vi "2013_01_02 Durability8 Main.vi"() -> ()   [LabVIEW 2011]
uses:
  MotorTypeDef.ctl
  <vilib>/DAQmx/write.llb/DAQmx Write (Counter Time 1Chan 1Samp).vi
  <vilib>/DAQmx/read.llb/DAQmx Read (Analog 1D Wfm NChan NSamp).vi
  <vilib>/Utility/TradDaqScaling.llb/Convert Thermistor Reading (waveform).vi
  <vilib>/DAQmx/miscellaneous.llb/DAQmx Fill In Error Info.vi
  <vilib>/measure/madcrms.llb/Averaged DC-RMS for N Chan.vi
  <vilib>/measure/NI_MAPro.lvlib
panel:
  out "for loop":i32
  out "Saving Data 2":bool caption="Saving Data"
  in  "new_file event":bool caption="new_file"
  out "Saving Data":bool
  in  "Coarse File Path":path=path "Durability/coarse.lvm"
  in  "Fine File Path":path=path "Durability/fine.lvm"
  out "Voltages":waveform(dbl)[](graph)
  out "Currents":waveform(dbl)[](graph)
  in  "Motor 8":T1 {"Elapsed Time" format="%<%H:%M:%S>t"; "Efficiency" format="%#_3g%%"; "Supply Voltage (V)" format="%#_3f"; "Power Output (W)" format="%#_3g"; "Power Usage (W)" format="%#_3g"; "Torque (mNm)" format="%#_3g"; "RPM" scale=0.0..40000.0 scale format="%#.6p"}
  in  "Motor 7":T1 {"Elapsed Time" format="%<%H:%M:%S>t"; "Efficiency" format="%#_3g%%"; "Supply Voltage (V)" format="%#_3f"; "Power Output (W)" format="%#_3g"; "Power Usage (W)" format="%#_3g"; "Torque (mNm)" format="%#_3g"; "RPM" scale=0.0..40000.0 scale format="%#.6p"}
  in  "Motor 6":T1 {"Elapsed Time" format="%<%H:%M:%S>t"; "Efficiency" format="%#_3g%%"; "Supply Voltage (V)" format="%#_3f"; "Power Output (W)" format="%#_3g"; "Power Usage (W)" format="%#_3g"; "Torque (mNm)" format="%#_3g"; "RPM" scale=0.0..40000.0 scale format="%#.6p"}
  in  "Motor 5":T1 {"Elapsed Time" format="%<%H:%M:%S>t"; "Efficiency" format="%#_3g%%"; "Supply Voltage (V)" format="%#_3f"; "Power Output (W)" format="%#_3g"; "Power Usage (W)" format="%#_3g"; "Torque (mNm)" format="%#_3g"; "RPM" scale=0.0..40000.0 scale format="%#.6p"}
  in  "Motor 4":T1 {"Elapsed Time" format="%<%H:%M:%S>t"; "Efficiency" format="%#_3g%%"; "Supply Voltage (V)" format="%#_3f"; "Power Output (W)" format="%#_3g"; "Power Usage (W)" format="%#_3g"; "Torque (mNm)" format="%#_3g"; "RPM" scale=0.0..40000.0 scale format="%#.6p"}
  in  "Motor 3":T1 {"Elapsed Time" format="%<%H:%M:%S>t"; "Efficiency" format="%#_3g%%"; "Supply Voltage (V)" format="%#_3f"; "Power Output (W)" format="%#_3g"; "Power Usage (W)" format="%#_3g"; "Torque (mNm)" format="%#_3g"; "RPM" scale=0.0..40000.0 scale format="%#.6p"}
  in  "Motor 2":T1 {"Elapsed Time" format="%<%H:%M:%S>t"; "Efficiency" format="%#_3g%%"; "Supply Voltage (V)" format="%#_3f"; "Power Output (W)" format="%#_3g"; "Power Usage (W)" format="%#_3g"; "Torque (mNm)" format="%#_3g"; "RPM" scale=0.0..40000.0 scale format="%#.6p"}
  in  "Motor 1":T1 {"Elapsed Time" format="%<%H:%M:%S>t"; "Efficiency" format="%#_3g%%"; "Supply Voltage (V)" format="%#_3f"; "Power Output (W)" format="%#_3g"; "Power Usage (W)" format="%#_3g"; "Torque (mNm)" format="%#_3g"; "RPM" scale=0.0..40000.0 scale format="%#.6p"}
  out "Motor Temp":dbl(slide) scale=90.0..110.0
  out "Tank Temp":dbl(slide) scale=90.0..110.0
  out "RMS Voltages":waveform(dbl)[](graph)
  out "RMS Currents":waveform(dbl)[](graph)
  in  "Temp Probe\nOn Motor":dbl=1.0
  out "loop time (ms)":u32
  in  "stop":bool
  in  "Unlock PWM":bool=TRUE
  in  "PWM 2":dbl(slide)=100.0 min=0.0 max=100.0 step=5.0 scale=0.0..100.0
  in  "PWM 1":dbl(slide) min=0.0 max=100.0 step=5.0 scale=0.0..100.0
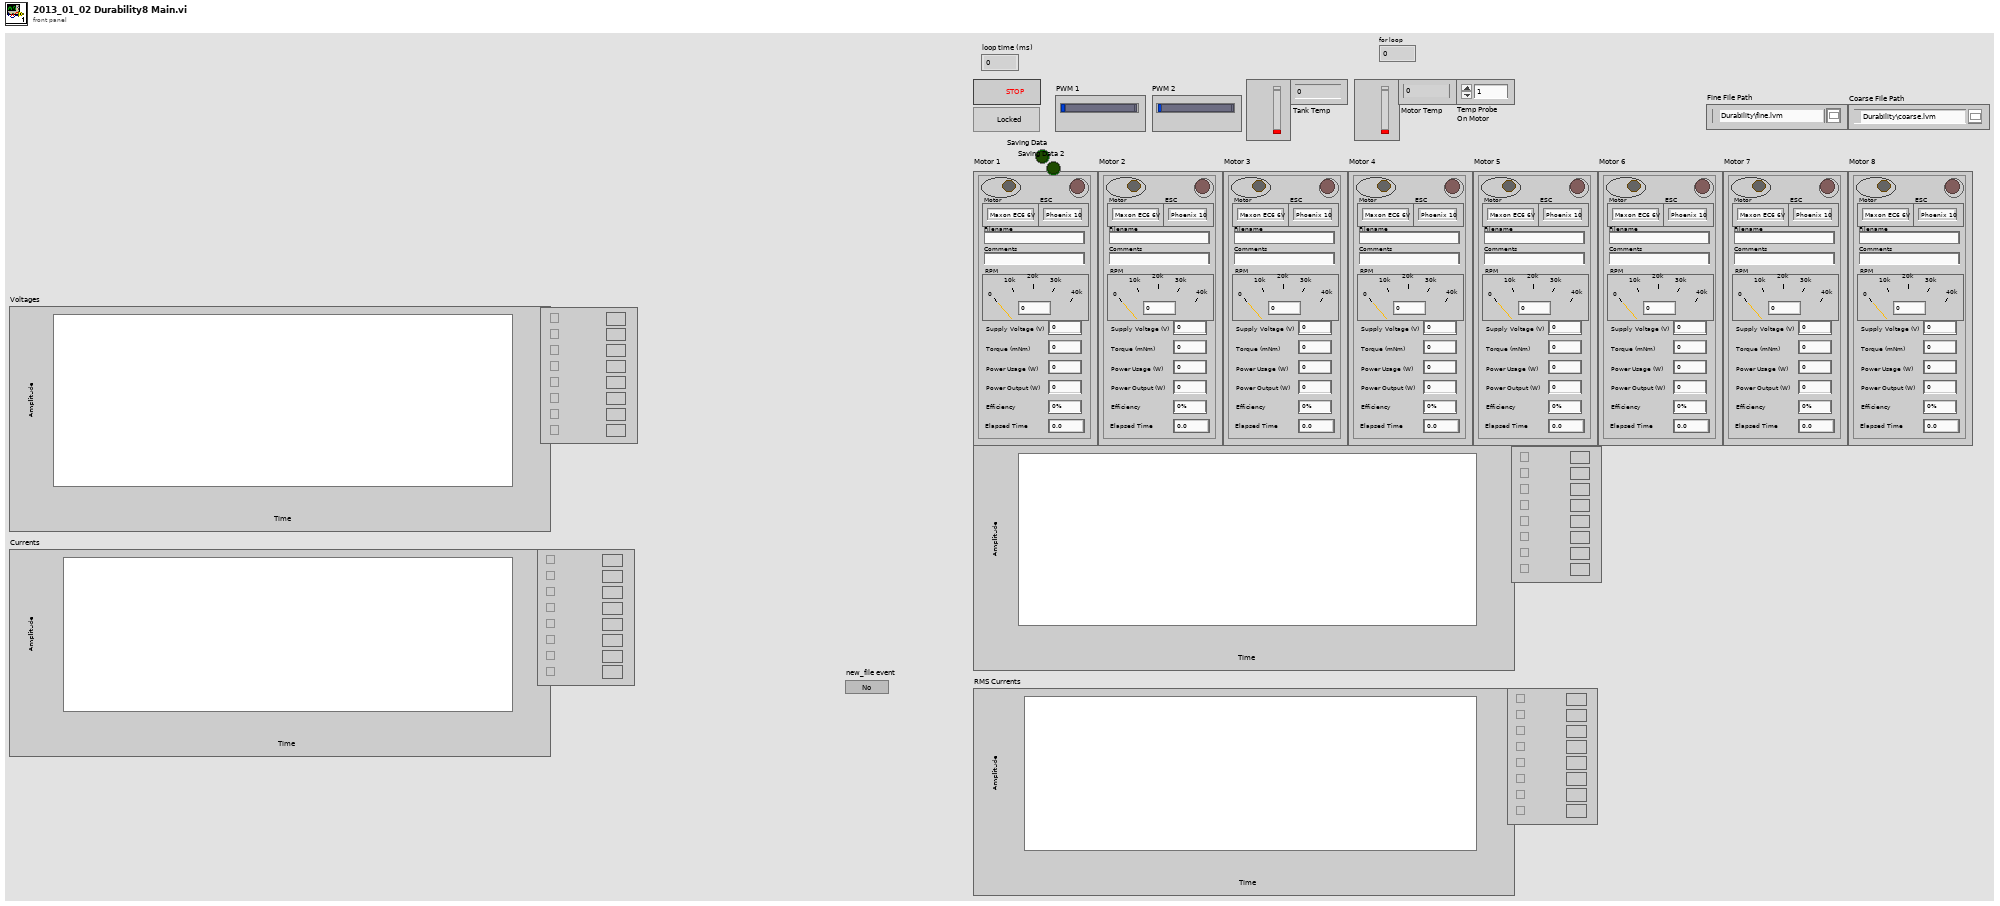
[diagram p1: front panel]
types:
  T1 = typedef "MotorTypeDef.ctl" = cluster{"Enabled":bool, "Fail":bool, "RPM":dbl, "Motor":enum16{"Maxon EC6 6V", "Maxon EC4 6V", "FH 0620 6V", "FH 0620 12V"}, "ESC":enum16{"Phoenix 10", "Maxon", "FH 1801"}, "Torque (mNm)":dbl, "Power Usage (W)":dbl, "Power Output (W)":dbl, "Supply Voltage (V)":dbl, "Efficiency":dbl, "Filename":string, "Comments":string, "Elapsed Time":dbl}
  T2 = enum8{"Enabled", "Disabled", "Disabled and Grayed Out"}
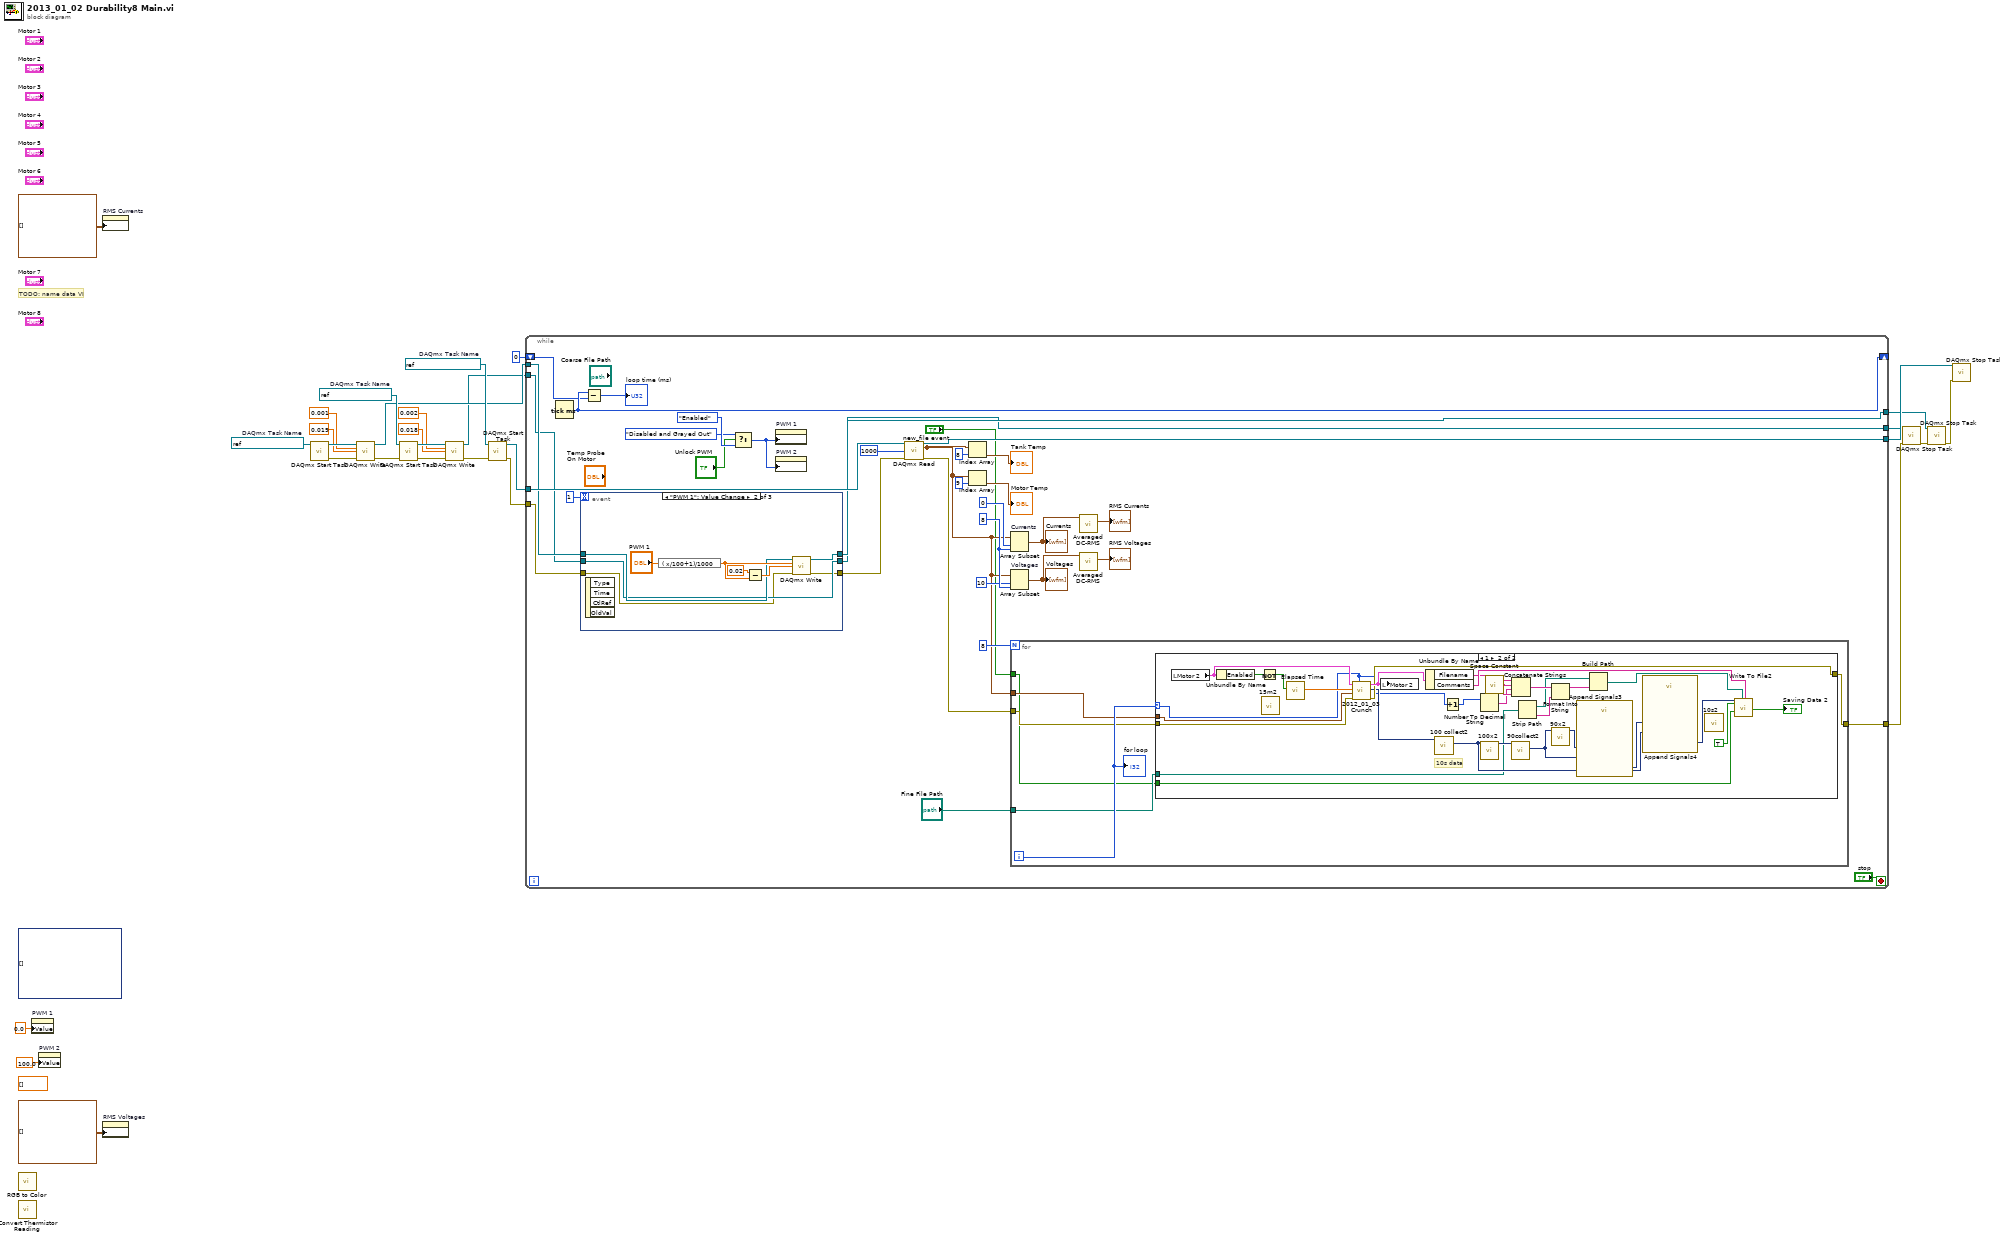
[diagram p0: block diagram]
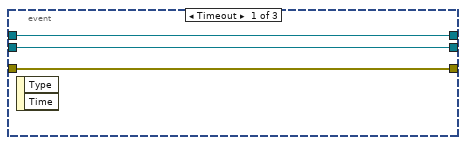
[diagram p2: hidden frame]
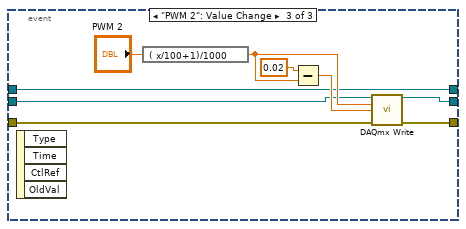
[diagram p3: hidden frame]
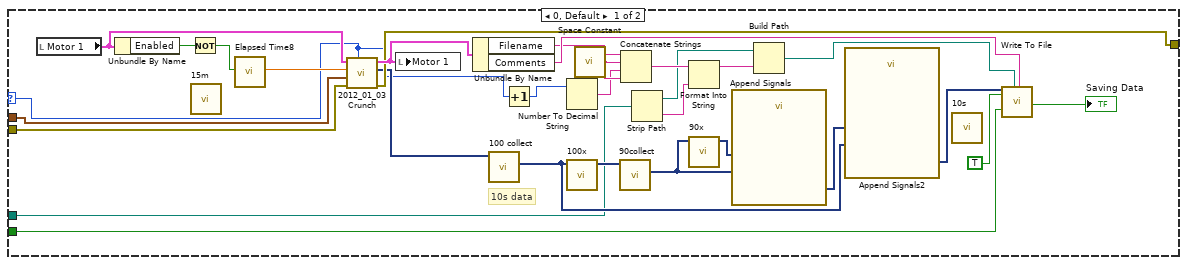
[diagram p4: hidden frame]
diagram:
  (unwired) dynamicdata[] []
  (unwired) dbl[] [] ("History Data")
  w23 = refnum<k21> "Durability8 PWM2"  # DAQmx Task Name
  w24 = refnum<k21> "Durability8 PWM1"  # DAQmx Task Name
  w28 = refnum<k21> "Durability8 Acquire"  # DAQmx Task Name
  # "TODO: name data VI"
  n1 = call <vilib>:"RGB to Color.vi"() -> ()  [unwired: 3 in, 1 out]
  n2 = call-poly <vilib>:"Convert Thermistor Reading.vi"() -> ()  [unwired: 7 in, 1 out]
  n3 = property on="PWM 1" class="Slide (strict)"("Value"=0.0 ("PWM 1")) -> ()  [unwired: 2 in, 2 out]
  n4 = property on="PWM 2" class="Slide (strict)"("Value"=100.0 ("PWM 2")) -> ()  [unwired: 2 in, 2 out]
  n5 = property on="RMS Currents" class="WFChart (strict)"("History Data"=waveform(dbl)[][] []) -> ()  [unwired: 2 in, 2 out]
  n6 = property on="RMS Voltages" class="WFChart (strict)"("History Data"=waveform(dbl)[][] []) -> ()  [unwired: 2 in, 2 out]
  n7 = call <vilib>:"DAQmx Start Task.vi"("task/channels in"=w24) -> ("task out"=w20:refnum<k21>, "error out"=w18:errorcluster)  [unwired: 13 in]
  n8 = call-poly <vilib>:"DAQmx Write.vi"("task/channels in"=w20, "high time"=0.001 ("data"), "low time"=0.019 ("data"), "error in"=w18) -> ("task out"=w22:refnum<k21>, "error out"=w17:errorcluster)  [unwired: 9 in, 1 out]
  n9 = call <vilib>:"DAQmx Start Task.vi"("task/channels in"=w23, "error in"=w17) -> ("task out"=w19:refnum<k21>, "error out"=w16:errorcluster)  [unwired: 12 in]
  n10 = call-poly <vilib>:"DAQmx Write.vi"("task/channels in"=w19, "high time"=0.002 ("data"), "low time"=0.018 ("data"), "error in"=w16) -> ("task out"=w21:refnum<k21>, "error out"=w15:errorcluster)  [unwired: 9 in, 1 out]
  n11 = call <vilib>:"DAQmx Start Task.vi"("task/channels in"=w28, "error in"=w15) -> ("task out"=w27:refnum<k21>, "error out"=w25:errorcluster)  [unwired: 12 in]
  n12 = while {
    tunnel: w27 -> [w63]
    tunnel: [w62] -> w26
    tunnel: w25 -> [w39]
    shift-right: [w56] -> _
    shift-left: u32 0 ("millisecond timer value") -> [w55]
    tunnel: w22 -> [w41]
    tunnel: w21 -> [w40]
    tunnel: [w38] -> w14
    tunnel: [w37] -> w5
    tunnel: [w29] -> w1
    stop <- "stop" stop-if-true
    w51 = 8 ("length")
    n13 = Tick Count (ms)() -> (millisecond timer value=w56:u32)
    n14 = event shown="[1] \"PWM 1\": Value Change" {
      selector: _ -> [_ _ _]
      dyn-events: _ -> [_ _ _]
      timeout: 1 -> [_ _ _]
      tunnel: w41 -> [w66 w71 w77]
      tunnel: w40 -> [w65 w69 w76]
      tunnel: [w66 w70 w77] -> w38
      tunnel: [w65 w69 w78] -> w37
      tunnel: [w64 w68 w79] -> w33
      tunnel: w39 -> [w64 w67 w80]
      event Timeout {
        n15 = event-data() -> ()  [unwired: 1 in, 2 out]
      }
      event "PWM 1": Value Change {
        n16 = event-data() -> ()  [unwired: 1 in, 4 out]
        n17 = expression code="( x/100+1)/1000"("PWM 1") -> (w72:dbl)
        n18 = Subtract(x=0.02 ("y"), y=w72) -> (x-y=w73:dbl)
        n19 = call-poly <vilib>:"DAQmx Write.vi"("task/channels in"=w71, "high time"=w72, "low time"=w73, "error in"=w67) -> ("task out"=w70:refnum<k21>, "error out"=w68:errorcluster)  [unwired: 9 in, 1 out]
      }
      event "PWM 2": Value Change {
        n20 = event-data() -> ()  [unwired: 1 in, 4 out]
        n21 = expression code="( x/100+1)/1000"("PWM 2") -> (w84:dbl)
        n22 = Subtract(x=0.02, y=w84) -> (x-y=w82:dbl)
        n23 = call-poly <vilib>:"DAQmx Write.vi"("task/channels in"=w76, "high time"=w84, "low time"=w82, "error in"=w80) -> ("task out"=w78:refnum<k21>, "error out"=w79:errorcluster)  [unwired: 9 in, 1 out]
      }
    }
    n24 = Subtract(x=w56, y=w55) -> (x-y=→"loop time (ms)":u32)
    n25 = Select(t=T2."Disabled and Grayed Out" ("Disabled"), s="Unlock PWM", f=T2."Enabled" ("Disabled")) -> (s? t:f=w60:T2)
    n26 = property on="PWM 1" class="Slide (strict)"("DisabledEnum"=w60) -> ()  [unwired: 2 in, 2 out]
    n27 = property on="PWM 2" class="Slide (strict)"("DisabledEnum"=w60) -> ()  [unwired: 2 in, 2 out]
    n28 = call-poly <vilib>:"DAQmx Read.vi"("task/channels in"=w63, "number of samples per channel"=1000, "error in"=w33) -> ("task out"=w62:refnum<k21>, "data"=w43:waveform(dbl)[], "error out"=w32:errorcluster)  [unwired: 10 in]
    n29 = Index Array(array=w43, index=8) -> (element=→"Tank Temp":waveform(dbl))
    n30 = Index Array(array=w43, index=9) -> (element=→"Motor Temp":waveform(dbl))
    n31 = Array Subset "Currents"(array=w43, index=0, length=w51) -> (w35:waveform(dbl)[])
    "Currents" <- w35
    n32 = Array Subset "Voltages"(array=w43, index=10 ("length"), length=w51) -> (w34:waveform(dbl)[])
    "Voltages" <- w34
    n33 = for {
      N: 8 -> [_]
      tunnel: w43 -> [w89]
      tunnel: w32 -> [w88]
      tunnel: "Fine File Path" -> [w87]
      tunnel: "new_file event" -> [w86]
      tunnel: [w85] -> w29
      i -> [w90]
      n34 = case shown="1" w90 {
        selector: w90 -> [w91 w121]
        tunnel: w89 -> [w96 w126]
        tunnel: w88 -> [w95 w125]
        tunnel: w87 -> [w99 w129]
        tunnel: w86 -> [w98 w128]
        tunnel: [w94 w124] -> w85
        frame 0, Default {
          # "10s data"
          n35 = local read "Motor 1"() -> (w118:T1)
          n36 = Unbundle By Name(w118) -> ("Enabled"=w120:bool)
          n37 = Not(x=w120) -> (.not. x?=w119:bool)
          n38 = call "15m"() -> ()  [unwired: 12 in, 8 out]
          n39 = call "Elapsed Time8"("Reset"=w119) -> ("Elapsed Time (s)"=w97:dbl)  [unwired: 11 in, 7 out]
          n40 = call "2012_01_03 Crunch.vi"("Numeric Control"=w91, "error in (no error)"=w95, "data"=w96, "Elapsed Time (s)"=w97, "Motor 8"=w118) -> ("error out"=w94:errorcluster, "Dynamic Data Type"=w93:dynamicdata, "Motor 9"=w102:T1)  [unwired: 4 in]
          n41 = local write "Motor 1"(w102) -> ()
          n42 = Unbundle By Name(w102) -> ("Filename"=w100:string, "Comments"=w101:string)
          n43 = call "100 collect"("Signals"=w93) -> ("Collected Signals"=w116:dynamicdata)  [unwired: 9 in, 1 out]
          n44 = Increment(x=w91) -> (x+1=w92:i32)
          n45 = Number To Decimal String(number=w92) -> (decimal integer string=w108:string)  [unwired: 1 in]
          n46 = call "100x"("Signals"=w116) -> ("Mean"=w112:dynamicdata)  [unwired: 8 in, 2 out]
          n47 = call <vilib>:"Space Constant.vi"() -> ("String"=w109:string)
          n48 = call "90collect"("Signals"=w112) -> ("Collected Signals"=w114:dynamicdata)  [unwired: 9 in, 1 out]
          n49 = Concatenate Strings(w100, w109, w108, w109) -> (w110:string)
          n50 = Strip Path(path=w99) -> (stripped path=w106:path, name=w107:string)
          n51 = Format Into String(initial string=w110, w107) -> (resulting string=w105:string)  [unwired: 2 in, 1 out]
          n52 = call "90x"("Signals"=w114) -> ("Mean"=w113:dynamicdata)  [unwired: 8 in, 2 out]
          n53 = call "Append Signals"("Input Signal B"=w114, "Input Signal A"=w113) -> ("Appended Signals"=w115:dynamicdata)  [unwired: 8 in, 1 out]
          n54 = Build Path(base path=w106, name or relative path=w105) -> (appended path=w111:path)
          n55 = call "Append Signals2"("Input Signal B"=w116, "Input Signal A"=w115) -> ("Appended Signals"=w117:dynamicdata)  [unwired: 8 in, 1 out]
          n56 = call "10s"() -> ()  [unwired: 12 in, 8 out]
          n57 = call "Write To File"("Signals"=w117, "Reset"=TRUE, "new_file"=w98, "Filename"=w111, "Comment"=w101) -> ("Saving Data"=→"Saving Data":bool)  [unwired: 12 in, 2 out]
        }
        frame 1 {
          # "10s data"
          n58 = local read "Motor 2"() -> (w148:T1)
          n59 = Unbundle By Name(w148) -> ("Enabled"=w150:bool)
          n60 = Not(x=w150) -> (.not. x?=w149:bool)
          n61 = call "15m2"() -> ()  [unwired: 12 in, 8 out]
          n62 = call "Elapsed Time"("Reset"=w149) -> ("Elapsed Time (s)"=w127:dbl)  [unwired: 11 in, 7 out]
          n63 = call "2012_01_03 Crunch.vi"("Numeric Control"=w121, "error in (no error)"=w125, "data"=w126, "Elapsed Time (s)"=w127, "Motor 8"=w148) -> ("error out"=w124:errorcluster, "Dynamic Data Type"=w123:dynamicdata, "Motor 9"=w132:T1)  [unwired: 4 in]
          n64 = local write "Motor 2"(w132) -> ()
          n65 = Unbundle By Name(w132) -> ("Filename"=w130:string, "Comments"=w131:string)
          n66 = call "100 collect2"("Signals"=w123) -> ("Collected Signals"=w146:dynamicdata)  [unwired: 9 in, 1 out]
          n67 = Increment(x=w121) -> (x+1=w122:i32)
          n68 = Number To Decimal String(number=w122) -> (decimal integer string=w138:string)  [unwired: 1 in]
          n69 = call "100x2"("Signals"=w146) -> ("Mean"=w142:dynamicdata)  [unwired: 8 in, 2 out]
          n70 = call <vilib>:"Space Constant.vi"() -> ("String"=w139:string)
          n71 = call "90collect2"("Signals"=w142) -> ("Collected Signals"=w144:dynamicdata)  [unwired: 9 in, 1 out]
          n72 = Concatenate Strings(w130, w139, w138, w139) -> (w140:string)
          n73 = Strip Path(path=w129) -> (stripped path=w136:path, name=w137:string)
          n74 = Format Into String(initial string=w140, w137) -> (resulting string=w135:string)  [unwired: 2 in, 1 out]
          n75 = call "90x2"("Signals"=w144) -> ("Mean"=w143:dynamicdata)  [unwired: 8 in, 2 out]
          n76 = call "Append Signals3"("Input Signal B"=w144, "Input Signal A"=w143) -> ("Appended Signals"=w145:dynamicdata)  [unwired: 8 in, 1 out]
          n77 = Build Path(base path=w136, name or relative path=w135) -> (appended path=w141:path)
          n78 = call "Append Signals4"("Input Signal B"=w146, "Input Signal A"=w145) -> ("Appended Signals"=w147:dynamicdata)  [unwired: 8 in, 1 out]
          n79 = call "10s2"() -> ()  [unwired: 12 in, 8 out]
          n80 = call "Write To File2"("Signals"=w147, "Reset"=TRUE, "new_file"=w128, "Filename"=w141, "Comment"=w131) -> ("Saving Data"=→"Saving Data 2":bool)  [unwired: 12 in, 2 out]
        }
      }
      "for loop" <- w90
    }
    n81 = call-poly <vilib>:"Averaged DC-RMS.vi"("signals in"=w35) -> ("RMS value waveforms"=→"RMS Currents":waveform(dbl)[])  [unwired: 6 in, 4 out]
    n82 = call-poly <vilib>:"Averaged DC-RMS.vi"("signals in"=w34) -> ("RMS value waveforms"=→"RMS Voltages":waveform(dbl)[])  [unwired: 6 in, 4 out]
  }
  n83 = call <vilib>:"DAQmx Stop Task.vi"("task/channels in"=w5, "error in"=w1) -> ("error out"=w13:errorcluster)  [unwired: 12 in, 1 out]
  n84 = call <vilib>:"DAQmx Stop Task.vi"("task/channels in"=w14, "error in"=w13) -> ("error out"=w12:errorcluster)  [unwired: 12 in, 1 out]
  n85 = call <vilib>:"DAQmx Stop Task.vi"("task/channels in"=w26, "error in"=w12) -> ()  [unwired: 12 in, 2 out]
